vi "LED_Brightness_Controller.vi"() -> ()   [LabVIEW 2021]
uses:
  <vilib>/Instr/_visa.llb/VISA Configure Serial Port (Instr).vi
panel:
  in  "Baud Rate (Bits/s)":u32(ring) items=["1200"=1200, "9600"=9600, "115200"=115200, "921600"=921600]
  in  "Stop Bits":u16(ring)=10 items=["1.0"=10, "2.0"=20]
  in  "Parity (0:none)":u16(ring) items=["None", "Odd", "Even"]
  in  "Word Length (Bits)":u16(ring) items=["8"=8, "9"=9]
  in  "VISA Resource input":refnum<visa-resource-name>
  in  "Stop Button":bool
  in  "SET Button":bool
  in  "Horizontal Pointer Slide":u8(slide)=1 caption="Brightness" max=100 step=10 scale=1.0..100.0
  # "LED_Brightness_Controller.vi\n\nPurpose:\nThis LabVIEW software provides an intuitive graphical interface for controlling the brightness of an LED via USART2. The user enters a percentage (0% to 100%) representing the desired brightness. The software sends this value to an STM32 microcontroller, which adjusts the LED's brightness by modifying the PWM duty cycle accordingly.\n\nFeatures:\n- Simple interface for setting LED brightness.\n- Real-time data transmission to the microcontroller via UART/USART.\n- Compatibility with the embedded C code provided in this repository.\n\nInstructions to Use the LabVIEW Software\nSteps:\n1. Install LabVIEW (compatible versions: [mention version if applicable]).\n2. Open the .vi file (LED_Brightness_Controller.vi) in LabVIEW.\n3. Set the correct COM port for your STM32 microcontroller in the VISA Resource input.\n4. Enter a brightness percentage (0–100%) in the designated input field.\n5. Press \"Send\" to transmit the brightness value via USART2.\n6. Observe the LED brightness change on your hardware.\n\nMohsen Anvari"
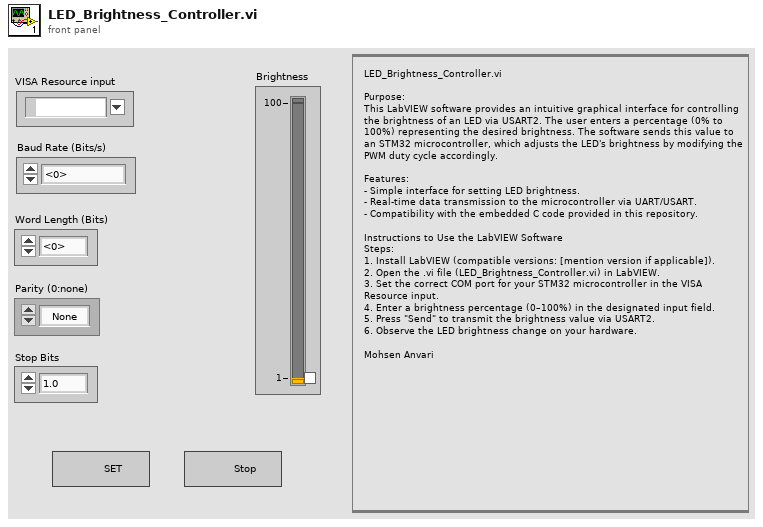
[diagram p1: front panel]
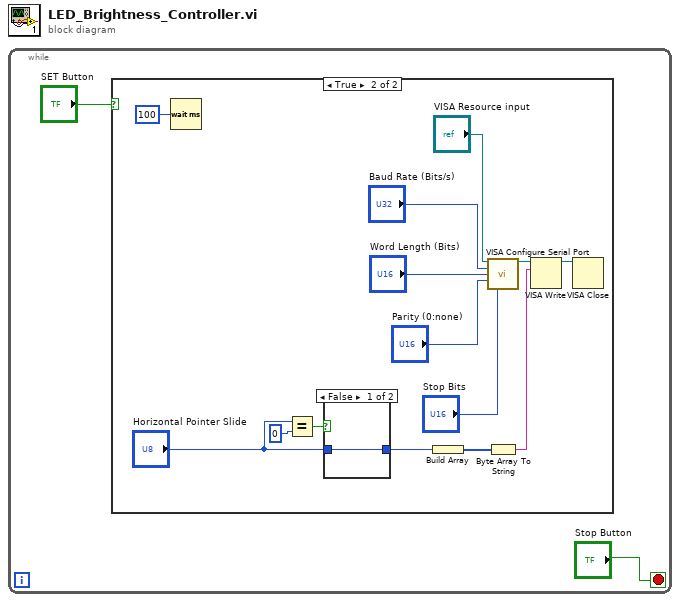
[diagram p0: block diagram]
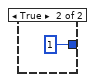
[diagram p3: hidden frame]
diagram:
  n1 = while {
    stop <- "Stop Button" stop-if-true
    n2 = case shown="True" "SET Button" {
      frame False {
      }
      frame True {
        n3 = Wait (ms)(milliseconds to wait=u32 100) -> ()  [unwired: 1 out]
        n4 = Equal?(x="Horizontal Pointer Slide", y=u8 0) -> (x = y?=w6:bool)
        n5 = case shown="False" w6 {
          tunnel: [w17 1] -> w5
          tunnel: "Horizontal Pointer Slide" -> [w17 _]
          frame False {
          }
          frame True {
          }
        }
        n6 = Build Array(w5) -> (w16:i32[])
        n7 = call-poly "VISA Configure Serial Port"("VISA resource name"="VISA Resource input", "baud rate (9600)"="Baud Rate (Bits/s)", "data bits (8)"="Word Length (Bits)", "parity (0:none)"="Parity (0:none)", "stop bits (10: 1 bit)"="Stop Bits") -> ("VISA resource name out"=w14:refnum<visa-resource-name>)  [unwired: 9 in, 1 out]
        n8 = Byte Array To String(unsigned byte array=w16) -> (string=w12:string)
        n9 = VISA Write(VISA resource name=w14, write buffer=w12) -> (VISA resource name out=w15:refnum<visa-resource-name>)  [unwired: 1 in, 2 out]
        n10 = VISA Close(VISA resource name=w15) -> ()  [unwired: 1 in, 1 out]
      }
    }
  }
